vi "Construct Tx.vi"(7 "error in (no error)":errorcluster, 9 "TX Parameters":T1={"channel #"=0, "channel handle"=0, "InstrumentHandle_board"=0, "InstrumentHandle_port"=0, "channel settings"={"Tx Board"=0, "Tx Port"=0, "Frame Array"=[], "QueueSizeIn"=1}} {"channel settings"."Frame Array"."Raw Frame" format="%.0x"; "channel settings"."Frame Array"."Frame Configuration"."interfaceID" format="%.0b"; "channel settings"."Frame Array"."HeaderInfo"."NetSelect" items=["FDX_TX_FRAME_DLY_A"=0, "FDX_TX_FRAME_DLY_B"=1, "FDX_TX_FRAME_BOTH "=3, "FDX_TX_FRAME_ONLY_A"=4, "FDX_TX_FRAME_ONLY_B "=5]; "channel settings"."Frame Array"."HeaderInfo"."FrameStartMode" items=["FDX_TX_FRAME_START_IFG", "FDX_TX_FRAME_START_PGWT", "FDX_TX_FRAME_START_TRG"]; "channel settings"."Frame Array"."HeaderInfo"."PhysErrorInjection" items=["FDX_TX_FRAME_ERR_OFF"=0, "FDX_TX_FRAME_ERR_CRC"=1, "FDX_TX_FRAME_ERR_ALI"=2, "FDX_TX_FRAME_ERR_PRE"=4, "FDX_TX_FRAME_ERR_PHY"=8]; "channel settings"."Frame Array"."HeaderInfo"."SequenceNumberInit" items=["FDX_TX_FRAME_SEQ_INIT_AUTO"=65535]; "channel settings"."Frame Array"."HeaderInfo"."SequenceNumberOffset" items=["FDX_TX_FRAME_SEQ_OFFS_AUTO "=65535]; "channel settings"."Frame Array"."HeaderInfo"."PayloadGenerationMode" items=["FDX_TX_FRAME_PGM_USER"=0, "FDX_TX_FRAME_PGM_IP_PART"=1, "FDX_TX_FRAME_PGM_IP_FULL"=2, "FDX_TX_FRAME_PGM_IP_PART_TT"=10, "FDX_TX_FRAME_PGM_IP_FULL_TT"=20]; "channel settings"."Frame Array"."HeaderInfo"."PayloadBufferMode" items=["FDX_TX_FRAME_PBM_STD", "FDX_TX_FRAME_PBM_MAC", "FDX_TX_FRAME_PBM_UDP"]}, 10 "Custom Device Ref In":T6=18446744073709551615 format="%.0x") -> (0 "error out":errorcluster, 2 "Tx Execution Unit out":refnum<class "Tx Generic Execution Unit.lvclass">, 3 "Custom Device Ref Out":T6=18446744073709551615 format="%.0x")   [LabVIEW 2020, in "AIM ARINC 664 Engine.lvlib" / "Implementation.lvlib" / "Tx Generic Execution Unit.lvclass"]
uses:
  Tx Generic Execution Unit.lvclass
  C:/repos/niveristand-aim-afdx-custom-device/Source/Custom Device Support/Engine/Implementation/Execution Unit/Execution Unit.lvclass
  <vilib>/NI VeriStand/Custom Device API/Custom Device Item Ref.ctl
  hardware_channels_tx.ctl
  channel_settings_tx.ctl
  Frame.ctl
  AIM LabVIEW src/src/_controls/queue_header_generic.ctl
  AIM LabVIEW src/src/_controls/queue_data_full.ctl
  Tx Generic Execution Unit.lvclass/Tx Generic Execution Unit.ctl
  Execution Unit Factory/Execution Unit Factory.lvclass
  Execution Unit/Execution Unit.lvclass
  <vilib>/NI VeriStand/Custom Device API/Custom Device API.lvlib
  AIM LabVIEW src/src/AIM664LV.lvlib
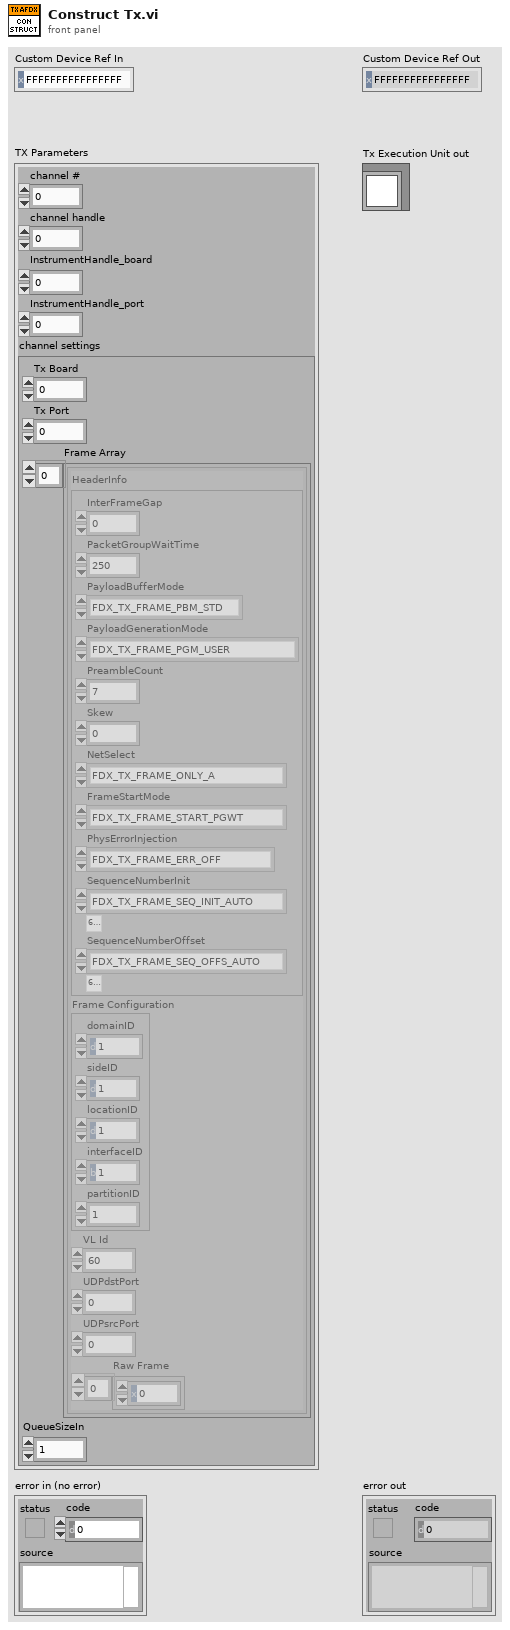
[diagram p1: front panel]
types:
  T1 = typedef "AIM ARINC 664 Engine.lvlib/Implementation.lvlib/Tx Generic Execution Unit.lvclass/hardware_channels_tx.ctl" = cluster{"channel #":u16, "channel handle":u64, "InstrumentHandle_board":u32, "InstrumentHandle_port":u32, "channel settings":T2}
  T2 = typedef "AIM ARINC 664 Engine.lvlib/Implementation.lvlib/Tx Generic Execution Unit.lvclass/channel_settings_tx.ctl" = cluster{"Tx Board":u32, "Tx Port":u32, "Frame Array":T3[], "QueueSizeIn":u32}
  T3 = typedef "Frame.ctl" = cluster{"HeaderInfo":T4, "Frame Configuration":T5, "VL Id":u16, "UDPdstPort":u16, "UDPsrcPort":u16, "Raw Frame":u8[]}
  T4 = typedef "AIM664LV.lvlib/queue_header_generic.ctl" = cluster{"InterFrameGap":u32, "PacketGroupWaitTime":u32, "PayloadBufferMode":u8, "PayloadGenerationMode":u8, "PreambleCount":u8, "Skew":u32, "NetSelect":u8, "FrameStartMode":u8, "PhysErrorInjection":u32, "SequenceNumberInit":u16, "SequenceNumberOffset":u16}
  T5 = typedef "AIM664LV.lvlib/queue_data_full.ctl" = cluster{"domainID":u8, "sideID":u8, "locationID":u8, "interfaceID":u8, "partitionID":u8}
  T6 = typedef "Custom Device API.lvlib/Custom Device Item Ref.ctl" = u64
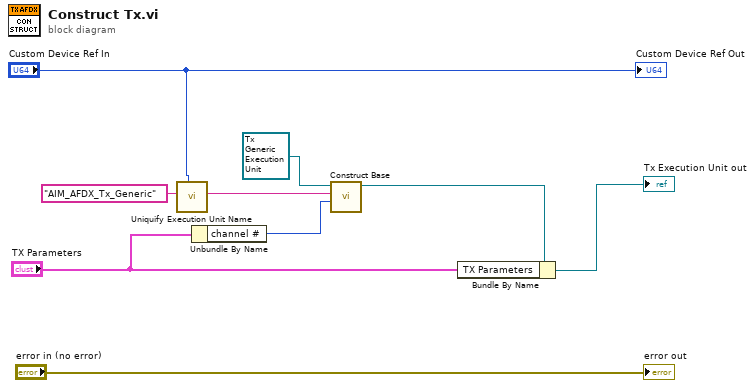
[diagram p0: block diagram]
diagram:
  n1 = call "Uniquify Execution Unit Name.vi"("custom device ref"="Custom Device Ref In", "execution unit name"="AIM_AFDX_Tx_Generic") -> ("execution unit name out"=w7:string)  [unwired: 9 in]
  n2 = Unbundle By Name("TX Parameters") -> ("channel #"=w6:u16)
  n3 = call "Construct Base.vi"("Execution Unit Implementation (default object)"=refnum<class "Tx Generic Execution Unit.lvclass"> refnum ("Communication Bus Template Interfaces:Implementation.lvlib:Tx Execution Unit.lvclass"), "identifier"=w7, "Channel"=w6) -> ("Execution Unit Out"=w4:refnum<class "Tx Generic Execution Unit.lvclass">)  [unwired: 6 in, 1 out]
  n4 = Bundle By Name(cluster=w4, "TX Parameters"="TX Parameters") -> (→"Tx Execution Unit out":refnum<class "Tx Generic Execution Unit.lvclass">)
  "error out" <- "error in (no error)"
  "Custom Device Ref Out" <- "Custom Device Ref In"
